vi "3.11-Critical Points V2.vi"(2 "Y (mm)":dbl[](array[numeric])=[-824.0, -821.8748054185536, -817.5016965016204, -818.8762184987505, -802.0414964088986, -800.9405372657634, -800.59012577146, -788.0816444032098, -786.2728465808068, -784.2245424325394, -781.9373558916932, -787.2650011250265, -784.474375788512, -778.521681763403, -776.2365810207972, -783.3658451204344, 730.5588889131224, 725.4102955430903, 724.8109075281693, 724.931328200215, 718.9384865393471, 714.6245895498994, 721.8640829579484, 720.0248002938554, 725.866494387571, 726.5437830014478, 731.9681149910491, 736.1878818898, 736.2022690917503, 745.9762624616667, 740.54860282115, 736.8877513302604, 737.0, -580.0, -600.0, -620.0, -640.0, -660.0, -680.0, -700.0, -720.0, -740.0, -760.0, -780.0, -800.0, -820.0, -840.0, -860.0, -880.0, -900.0, -920.0, -940.0, -960.0, -980.0, -1000.0, -1020.0, -1040.0, -1060.0, -1080.0, -1100.0, -1120.0, -1140.0, -1160.0, 580.0, 600.0, 620.0, 640.0, 660.0, 680.0, 700.0, 720.0, 740.0, 760.0, 780.0, 800.0, 820.0, 840.0, 860.0, 880.0, 900.0, 920.0, 940.0, 960.0, 980.0, 1000.0, 1020.0, 1040.0, 1060.0, 1080.0, 1100.0, 1120.0, 1140.0, 1160.0], 3 "X (mm)":dbl[](array[numeric])=[840.0, 854.3458780914469, 868.5477883026458, 882.9154841192139, 896.0842048902769, 910.0732171691171, 924.145412930461, 936.7642586636871, 950.5034421622921, 964.2089652419434, 977.8766530675427, 993.028814291989, 1006.7451760358431, 1019.7358924207481, 1033.5375164797342, 1049.9022455781442, 1049.4843904209192, 1034.373102871993, 1020.7156560129519, 1007.3635844318354, 992.8150927510532, 978.9089486341247, 967.2841142298599, 954.0407250143282, 942.0138830037281, 929.2083593725679, 916.9329489649929, 904.4080938905194, 891.4802776231645, 879.0949593134791, 865.8605270565532, 852.8624235442778, 840.0, 0.0, 0.0, 0.0, 0.0, 0.0, 0.0, 0.0, 0.0, 0.0, 0.0, 0.0, 0.0, 0.0, 0.0, 0.0, 0.0, 0.0, 0.0, 0.0, 0.0, 0.0, 0.0, 0.0, 0.0, 0.0, 0.0, 0.0, 0.0, 0.0, 0.0, 0.0, 0.0, 0.0, 0.0, 0.0, 0.0, 0.0, 0.0, 0.0, 0.0, 0.0, 0.0, 0.0, 0.0, 0.0, 0.0, 0.0, 0.0, 0.0, 0.0, 0.0, 0.0, 0.0, 0.0, 0.0, 0.0, 0.0, 0.0, 0.0, 0.0]) -> (0 "Left Data":T2, 1 "Right Data":T1)   [LabVIEW 2010]
uses:
  3.0-Global.vi
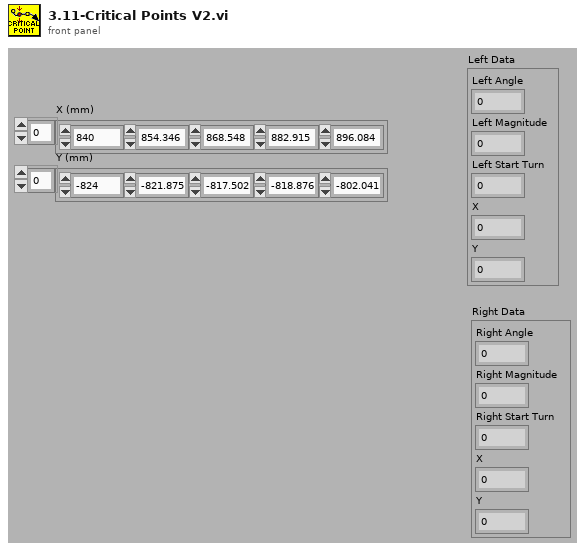
[diagram p1: front panel]
types:
  T1 = cluster{"Right Angle":dbl, "Right Magnitude":dbl, "Right Start Turn":dbl, "X":dbl, "Y":dbl}
  T2 = cluster{"Left Angle":dbl, "Left Magnitude":dbl, "Left Start Turn":dbl, "X":dbl, "Y":dbl}
  T3 = cluster{" Angle":dbl, " Magnitude":dbl, " Start Turn":dbl, "X":dbl, "Y":dbl}
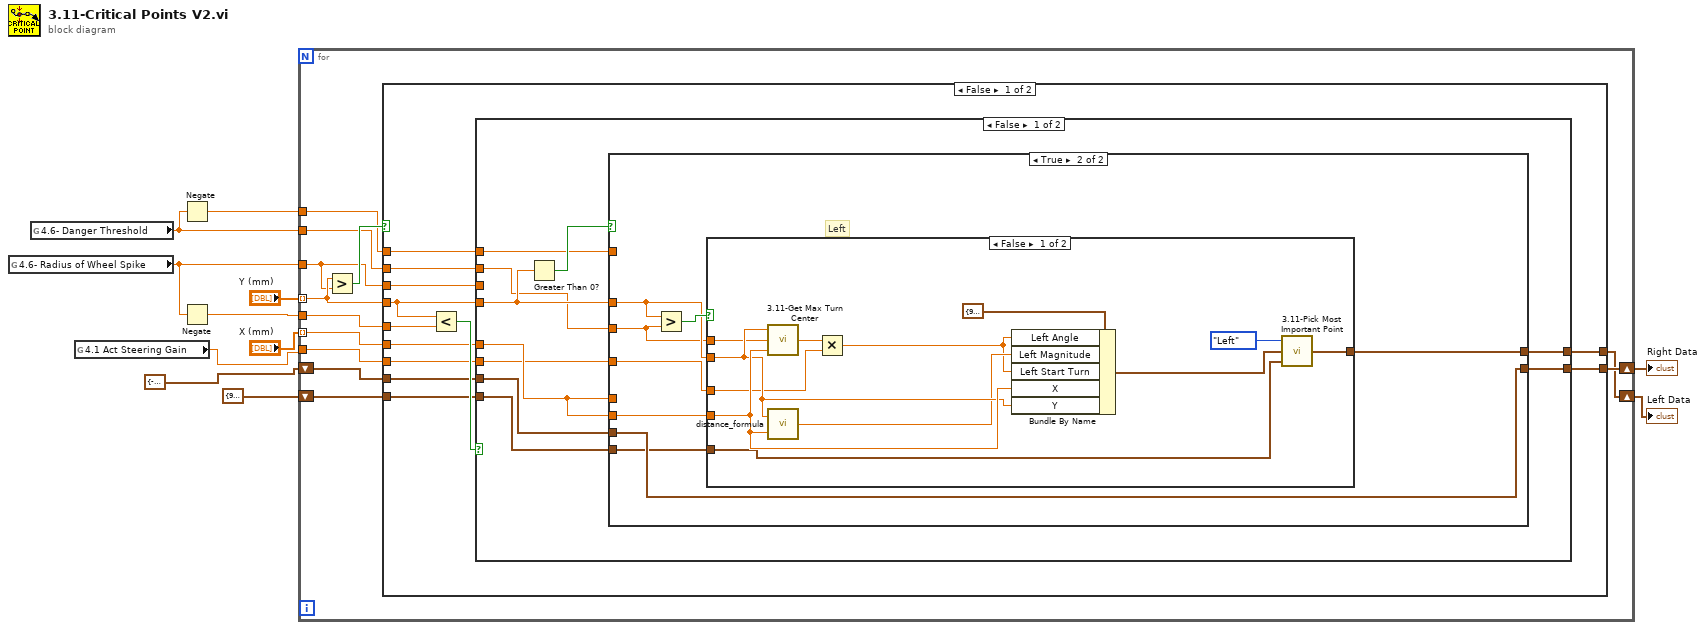
[diagram p0: block diagram]
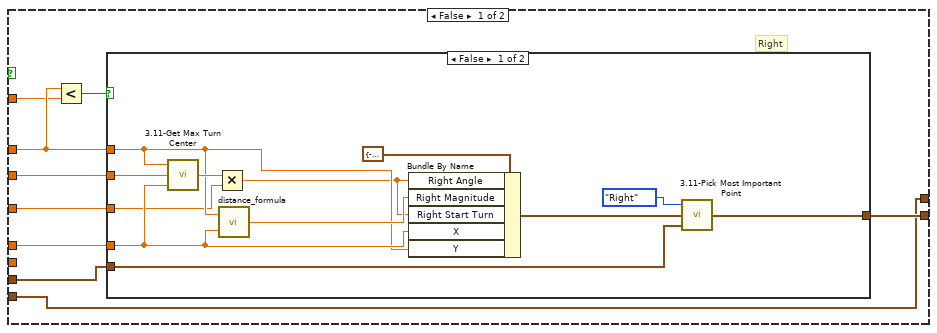
[diagram p2: hidden frame]
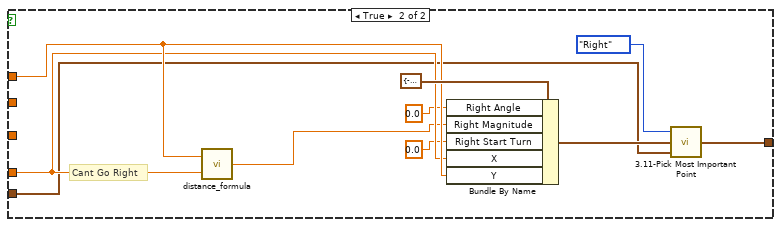
[diagram p3: hidden frame]
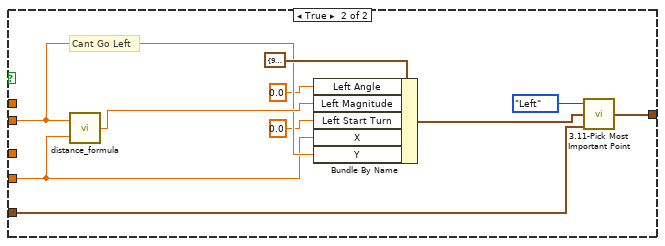
[diagram p4: hidden frame]
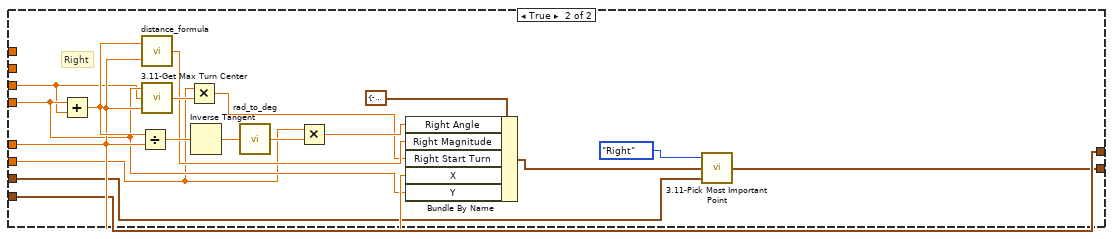
[diagram p5: hidden frame]
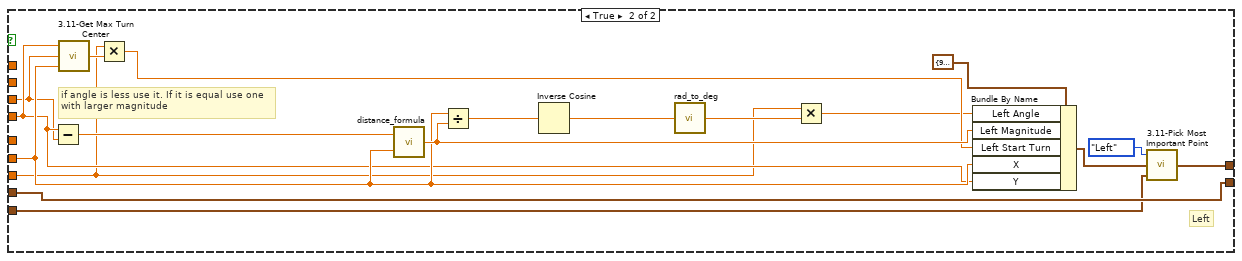
[diagram p6: hidden frame]
diagram:
  n1 = global read "3.0-Global.vi" "4.6- Radius of Wheel Spike"() -> (w5:dbl)
  n2 = global read "3.0-Global.vi" "4.6- Danger Threshold"() -> (w3:dbl)
  n3 = global read "3.0-Global.vi" "4.1 Act Steering Gain"() -> (w1:dbl)
  n4 = Negate(x=w3) -> (-x=w2:dbl)
  n5 = Negate(x=w5) -> (-x=w4:dbl)
  n6 = for {
    tunnel: "Y (mm)" -> [w22] mode=indexing
    tunnel: "X (mm)" -> [w21] mode=indexing
    shift-right: [w19] -> w9
    shift-left: T2 {"Left Angle"=90.0, "Left Magnitude"=0.0, "Left Start Turn"=90.0, "X"=-1.0, "Y"=0.0} ("input cluster") -> [w18]
    shift-right: [w20] -> w8
    shift-left: T1 {"Right Angle"=-90.0, "Right Magnitude"=0.0, "Right Start Turn"=-90.0, "X"=-1.0, "Y"=0.0} ("input cluster") -> [w17]
    tunnel: w5 -> [w15]
    tunnel: w4 -> [w16]
    tunnel: w3 -> [w14]
    tunnel: w2 -> [w13]
    tunnel: w1 -> [w12]
    n7 = Greater?(x=w22, y=w15) -> (0:w23:bool)
    n8 = case shown="False" w23 {
      tunnel: w22 -> [w33 w135]
      tunnel: w21 -> [w34 w136]
      tunnel: [w30 w133] -> w20
      tunnel: [w32 w131] -> w19
      tunnel: w18 -> [w31 w130]
      tunnel: w17 -> [w29 w133]
      tunnel: w16 -> [w28 _]
      tunnel: w15 -> [w27 w128]
      tunnel: w14 -> [w26 _]
      tunnel: w13 -> [w25 _]
      tunnel: w12 -> [w24 w125]
      frame False {
        n9 = Less?(x=w33, y=w28) -> (x < y?=w35:bool)
        n10 = case shown="False" w35 {
          tunnel: w34 -> [w43 w117]
          tunnel: w33 -> [w44 w116]
          tunnel: [w42 w113] -> w30
          tunnel: [w41 w115] -> w32
          tunnel: w31 -> [w39 w115]
          tunnel: w29 -> [w40 w112]
          tunnel: w27 -> [_ w110]
          tunnel: w26 -> [w38 _]
          tunnel: w25 -> [w37 _]
          tunnel: w24 -> [w36 w107]
          frame False {
            n11 = Greater Than 0?(x=w44) -> (x > 0?=w45:bool)
            n12 = case shown="True" w45 {
              tunnel: w44 -> [w53 w83]
              tunnel: w43 -> [_ w82]
              tunnel: w43 -> [w52 _]
              tunnel: [w51 w80] -> w42
              tunnel: [w50 w81] -> w41
              tunnel: w40 -> [w49 w80]
              tunnel: w39 -> [w50 w79]
              tunnel: w38 -> [w47 w78]
              tunnel: w37 -> [w48 _]
              tunnel: w36 -> [w46 w77]
              frame False {
                # "Right"
                n13 = Less?(x=w53, y=w48) -> (x < y?=w54:bool)
                n14 = case shown="False" w54 {
                  tunnel: w53 -> [w62 w75]
                  tunnel: w52 -> [w63 w74]
                  tunnel: [w58 w70] -> w51
                  tunnel: w49 -> [w60 w68]
                  tunnel: w47 -> [w57 _]
                  tunnel: w46 -> [w55 _]
                  frame False {
                    n15 = call "3.11-Get Max Turn Center.vi"("X (mm)"=w63, "Distance Along Y where polar system is centered"=w57, "Y (mm)"=w62) -> ("Start Turn Angle"=w65:dbl)
                    n16 = Multiply(x=w65, y=w55) -> (x*y=w56:dbl)
                    n17 = call "distance_formula.vi"("X2 - X1"=w63, "Y2 - Y1"=w62) -> ("Distance"=w64:dbl)
                    n18 = Bundle By Name(cluster=T1 {"Right Angle"=-90.0, "Right Magnitude"=0.0, "Right Start Turn"=-90.0, "X"=-1.0, "Y"=-1701.0} ("input cluster"), "Right Angle"=w56, "Right Magnitude"=w64, "Right Start Turn"=w56, "X"=w63, "Y"=w62) -> (w61:T1)
                    n19 = call "3.11-Pick Most Important Point.vi"("Old Point"=w60, "New Point"=w61, "Side"=enum16{"Left", "Right"}."Right") -> ("Most Limiting Point"=w58:T3)
                  }
                  frame True {
                    # "Cant Go Right"
                    n20 = call "distance_formula.vi"("X2 - X1"=w74, "Y2 - Y1"=w75) -> ("Distance"=w73:dbl)
                    n21 = Bundle By Name(cluster=T1 {"Right Angle"=-90.0, "Right Magnitude"=0.0, "Right Start Turn"=-90.0, "X"=-1.0, "Y"=-1701.0} ("input cluster"), "Right Angle"=0.0 ("y"), "Right Magnitude"=w73, "Right Start Turn"=0.0 ("y"), "X"=w74, "Y"=w75) -> (w69:T1)
                    n22 = call "3.11-Pick Most Important Point.vi"("Old Point"=w68, "New Point"=w69, "Side"=enum16{"Left", "Right"}."Right") -> ("Most Limiting Point"=w70:T3)
                  }
                }
              }
              frame True {
                # "Left"
                n23 = Greater?(x=w83, y=w78) -> (0:w84:bool)
                n24 = case shown="False" w84 {
                  tunnel: w83 -> [w94 w104]
                  tunnel: w82 -> [w95 w103]
                  tunnel: [w91 w100] -> w81
                  tunnel: w79 -> [w89 w98]
                  tunnel: w78 -> [w87 _]
                  tunnel: w77 -> [w85 _]
                  frame False {
                    n25 = call "3.11-Get Max Turn Center.vi"("X (mm)"=w95, "Distance Along Y where polar system is centered"=w87, "Y (mm)"=w94) -> ("Start Turn Angle"=w93:dbl)
                    n26 = call "distance_formula.vi"("X2 - X1"=w95, "Y2 - Y1"=w94) -> ("Distance"=w92:dbl)
                    n27 = Multiply(x=w93, y=w85) -> (x*y=w86:dbl)
                    n28 = Bundle By Name(cluster=T2 {"Left Angle"=90.0, "Left Magnitude"=0.0, "Left Start Turn"=90.0, "X"=-1.0, "Y"=1701.0} ("input cluster"), "Left Angle"=w86, "Left Magnitude"=w92, "Left Start Turn"=w86, "X"=w95, "Y"=w94) -> (w90:T2)
                    n29 = call "3.11-Pick Most Important Point.vi"("Old Point"=w89, "New Point"=w90, "Side"=enum16{"Left", "Right"}."Left") -> ("Most Limiting Point"=w91:T3)
                  }
                  frame True {
                    # "Cant Go Left"
                    n30 = call "distance_formula.vi"("X2 - X1"=w103, "Y2 - Y1"=w104) -> ("Distance"=w105:dbl)
                    n31 = Bundle By Name(cluster=T2 {"Left Angle"=90.0, "Left Magnitude"=0.0, "Left Start Turn"=90.0, "X"=-1.0, "Y"=1701.0} ("input cluster"), "Left Angle"=0.0 ("y"), "Left Magnitude"=w105, "Left Start Turn"=0.0 ("y"), "X"=w103, "Y"=w104) -> (w99:T2)
                    n32 = call "3.11-Pick Most Important Point.vi"("Old Point"=w98, "New Point"=w99, "Side"=enum16{"Left", "Right"}."Left") -> ("Most Limiting Point"=w100:T3)
                  }
                }
              }
            }
          }
          frame True {
            # "Right"
            n33 = Add(x=w116, y=w110) -> (x+y=w123:dbl)
            n34 = Divide(x=w123, y=w117) -> (x/y=w124:dbl)
            n35 = call "distance_formula.vi"("X2 - X1"=w117, "Y2 - Y1"=w123) -> ("Distance"=w118:dbl)
            n36 = call "3.11-Get Max Turn Center.vi"("X (mm)"=w117, "Distance Along Y where polar system is centered"=w110, "Y (mm)"=w116) -> ("Start Turn Angle"=w119:dbl)
            n37 = Multiply(x=w107, y=w119) -> (x*y=w108:dbl)
            n38 = Inverse Tangent(1:w124) -> (0:w120:dbl)
            n39 = call "rad_to_deg.vi"("Radians"=w120) -> ("Degrees"=w121:dbl)
            n40 = Multiply(x=w107, y=w121) -> (x*y=w109:dbl)
            n41 = Bundle By Name(cluster=T1 {"Right Angle"=-90.0, "Right Magnitude"=0.0, "Right Start Turn"=-90.0, "X"=-1.0, "Y"=-1701.0} ("input cluster"), "Right Angle"=w109, "Right Magnitude"=w118, "Right Start Turn"=w108, "X"=w117, "Y"=w116) -> (w114:T1)
            n42 = call "3.11-Pick Most Important Point.vi"("Old Point"=w112, "New Point"=w114, "Side"=enum16{"Left", "Right"}."Right") -> ("Most Limiting Point"=w113:T3)
          }
        }
      }
      frame True {
        # "if angle is less use it. If it is equal use one\nwith larger magnitude"
        # "Left"
        n43 = Subtract(x=w135, y=w128) -> (x-y=w142:dbl)
        n44 = call "3.11-Get Max Turn Center.vi"("X (mm)"=w136, "Distance Along Y where polar system is centered"=w128, "Y (mm)"=w135) -> ("Start Turn Angle"=w134:dbl)
        n45 = Multiply(x=w125, y=w134) -> (x*y=w127:dbl)
        n46 = call "distance_formula.vi"("X2 - X1"=w136, "Y2 - Y1"=w142) -> ("Distance"=w137:dbl)
        n47 = Divide(x=w136, y=w137) -> (x/y=w141:dbl)
        n48 = Inverse Cosine(1:w141) -> (0:w139:dbl)
        n49 = call "rad_to_deg.vi"("Radians"=w139) -> ("Degrees"=w138:dbl)
        n50 = Multiply(x=w125, y=w138) -> (x*y=w126:dbl)
        n51 = Bundle By Name(cluster=T2 {"Left Angle"=90.0, "Left Magnitude"=0.0, "Left Start Turn"=90.0, "X"=-1.0, "Y"=1701.0} ("input cluster"), "Left Angle"=w126, "Left Magnitude"=w137, "Left Start Turn"=w127, "X"=w136, "Y"=w135) -> (w132:T2)
        n52 = call "3.11-Pick Most Important Point.vi"("Old Point"=w130, "New Point"=w132, "Side"=enum16{"Left", "Right"}."Left") -> ("Most Limiting Point"=w131:T3)
      }
    }
  }
  "Left Data" <- w9
  "Right Data" <- w8
